vi "PathPlanner_EventMarker_Equals.vi"(9 "Other EventMarker":T1, 11 "EventMarker":T1) -> (3 "Equal":bool)   [LabVIEW 2019, in "PathPlanner24.lvlib"]
doc: "Determinesif two event markers are equal\n\nInputs:\n - EventMarker - cluster - Data cluster\n - OtherEventMarker - cluster - Data cluster\n\nOutputs:\n - Equal - boolean - TRUE if both event markers are equal"
uses:
  PathPlanner24.lvlib
  <vilib>/Rock Robotics/WPI/ThirdParty/JAS_Junk/TrajLib/Trajectory_Library.lvlib
  TypeDef/PathPlannerCommandUtil.ctl
  TypeDef/PathPlannerEventMarker.ctl
  ENum/PathPlanner_TrajectoryEvent_Type_ENUM.ctl
  ENum/PathPlanner_CommandUtil_Type_ENUM.ctl
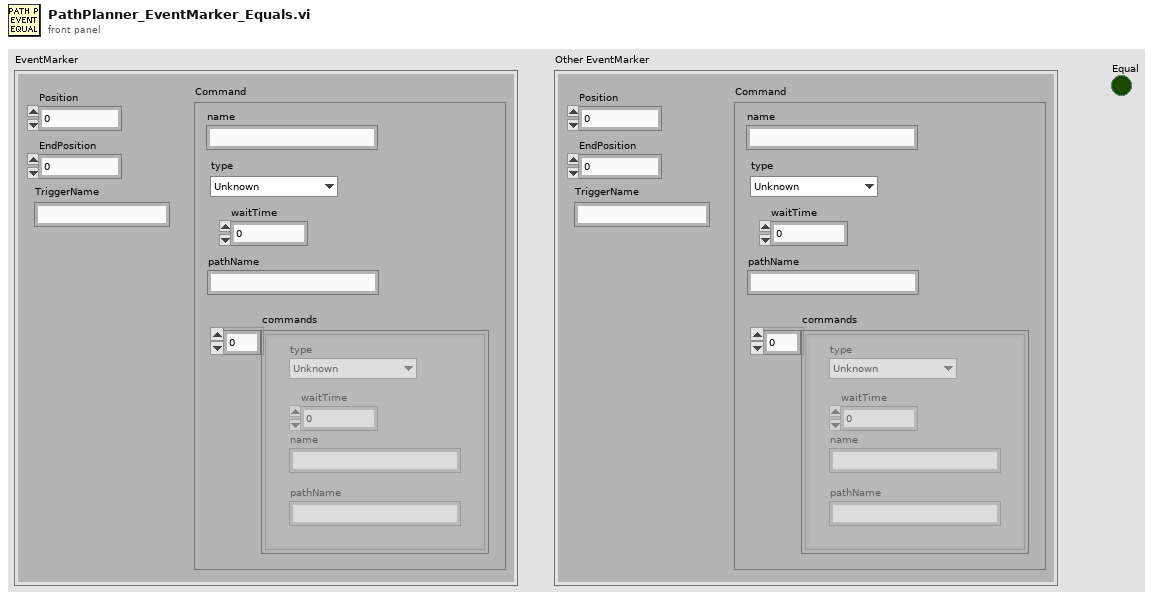
[diagram p1: front panel]
types:
  T1 = typedef "PathPlanner24.lvlib/PathPlannerEventMarker.ctl" = cluster{"Position":dbl, "Command":T2, "TriggerName":string, "EndPosition":dbl}
  T2 = typedef "PathPlanner24.lvlib/PathPlannerCommandUtil.ctl" = cluster{"waitTime":dbl, "name":string, "pathName":string, "commands":cluster{"type":T3, "waitTime":dbl, "name":string, "pathName":string}[], "type":T4}
  T3 = typedef "PathPlanner24.lvlib/PathPlanner_TrajectoryEvent_Type_ENUM.ctl" = enum16{"Unknown", "Wait", "Named", "Path", "Sequential", "Parallel", "Race", "Deadline", "PointTowardsZoneEnter", "PointTowardsZoneExit", "TriggerEventStart", "TriggerEventStop", "TriggerEventOneshot"}
  T4 = typedef "PathPlanner24.lvlib/PathPlanner_CommandUtil_Type_ENUM.ctl" = enum16{"Unknown", "Wait", "Named", "Path", "Sequential", "Parallel", "Race", "Deadline"}
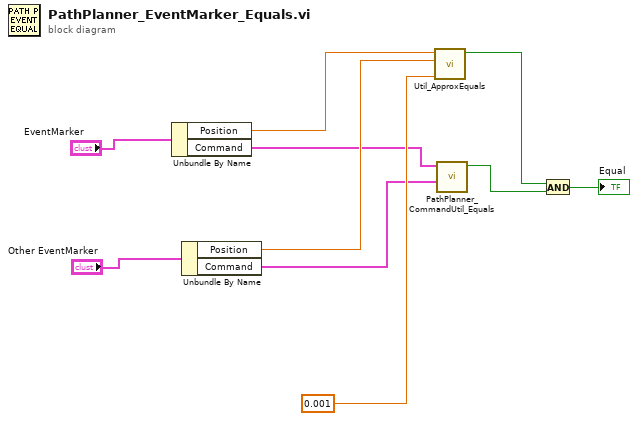
[diagram p0: block diagram]
diagram:
  n1 = Unbundle By Name("EventMarker") -> ("Position"=w6:dbl, "Command"=w3:T2)
  n2 = Unbundle By Name("Other EventMarker") -> ("Position"=w5:dbl, "Command"=w2:T2)
  n3 = call <vilib>:"Util_ApproxEquals.vi"("Tolerance"=0.001 ("y"), "Value 2"=w5, "Value 1"=w6) -> ("ApproxEquals"=w4:bool)  [unwired: 8 in]
  n4 = call "PathPlanner_CommandUtil_Equals.vi"("Other EventMarker"=w2, "Command"=w3) -> ("Equal"=w1:bool)  [unwired: 9 in]
  n5 = And(x=w4, y=w1) -> (x .and. y?=→"Equal":bool)
